vi "FlatToRichnixnet_grpc_DbFindObjectRequest.vi"(5 "OutputClusterType":T1, 11 "InputCluster":T3) -> (3 "OutputCluster":T1)   [LabVIEW 2025, in "grpc-xnet_client.lvlib"]
uses:
  nixnet_grpc_DbFindObjectRequest_Flat.ctl
  nidevice_grpc_Session_Flat.ctl
  nixnet_grpc_DbFindObjectRequest.ctl
  nidevice_grpc_Session.ctl
  grpc-xnet_client.lvlib
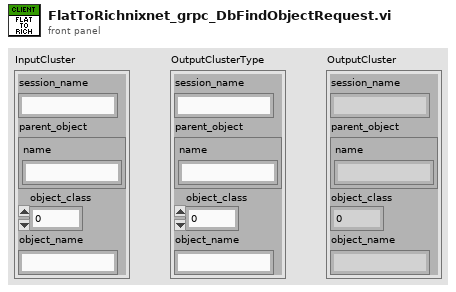
[diagram p1: front panel]
types:
  T1 = typedef "grpc-xnet_client.lvlib/nixnet_grpc_DbFindObjectRequest.ctl" = cluster{"session_name":string, "parent_object":T2, "object_class":u32, "object_name":string}
  T2 = typedef "grpc-xnet_client.lvlib/nidevice_grpc_Session.ctl" = cluster{"name":string}
  T3 = typedef "grpc-xnet_client.lvlib/nixnet_grpc_DbFindObjectRequest_Flat.ctl" = cluster{"session_name":string, "parent_object":T4, "object_class":u32, "object_name":string}
  T4 = typedef "grpc-xnet_client.lvlib/nidevice_grpc_Session_Flat.ctl" = cluster{"name":string}
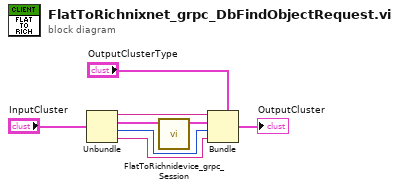
[diagram p0: block diagram]
diagram:
  n1 = Unbundle "Unbundle"("InputCluster") -> ("session_name"=w5:string, "parent_object"=w4:T4, "object_class"=w2:u32, "object_name"=w1:string)
  n2 = call "FlatToRichnidevice_grpc_Session.vi"("InputCluster"=w4) -> ("OutputCluster"=w3:T2)  [unwired: 10 in]
  n3 = Bundle "Bundle"(cluster="OutputClusterType", "session_name"=w5, "parent_object"=w3, "object_class"=w2, "object_name"=w1) -> (→"OutputCluster":T1)
